vi "Ball Posession Status.vi"(7 "Override?":bool, 9 "Logical Exit?":bool, 10 "Using Sensor?":bool, 11 "Sensor":bool) -> (3 "Ball Posessed?":bool)   [LabVIEW 2015]
uses:
  Common Code/Change Detect Boolean.vi
panel:
  in  "Override to True?":bool
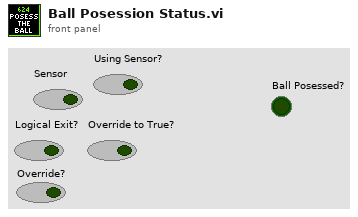
[diagram p1: front panel]
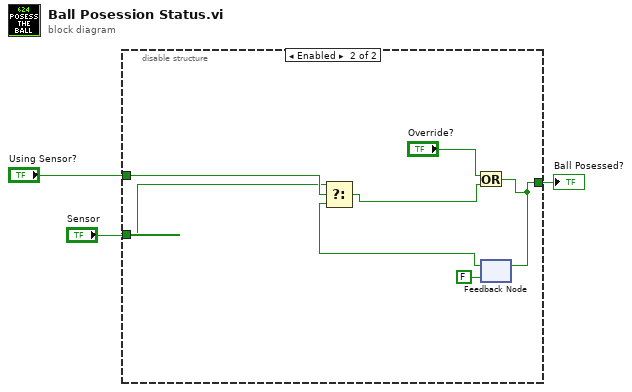
[diagram p0: block diagram]
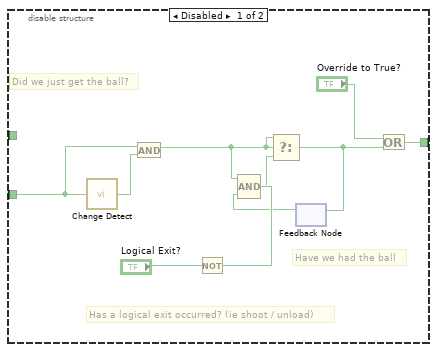
[diagram p2: hidden frame]
diagram:
  n1 = disable-structure shown="Enabled" {
    disable-tunnel: "Sensor" -> [w12 w19]
    disable-tunnel: [w6 w14] -> w2
    disable-tunnel: "Using Sensor?" -> [_ w20]
    frame Disabled {
      # "Has a logical exit occurred? (ie shoot / unload)"
      # "Have we had the ball"
      # "Did we just get the ball?"
      n2 = call-poly "Change Detect.vi"("In"=w12) -> ("Changed?"=w13:bool)
      n3 = And(x=w12, y=w13) -> (x .and. y?=w4:bool)
      n4 = Not(x="Logical Exit?") -> (.not. x?=w10:bool)
      n5 = feedback #1() -> (w9:bool)  [unwired: 1 in]
      n6 = Compound Arithmetic op=AND(w4, w10, w9) -> (w8:bool)
      n7 = Select(t=w4, s=w4, f=w8) -> (s? t:f=w7:bool)
      n8 = feedback-in #1(w7) -> ()
      n9 = Or(x="Override to True?", y=w7) -> (x .or. y?=w6:bool)
    }
    frame Enabled {
      n10 = feedback #2(FALSE ("Sensor")) -> (w17:bool)
      n11 = Select(t=w19, s=w20, f=w17) -> (s? t:f=w15:bool)
      n12 = Or(x="Override?", y=w15) -> (x .or. y?=w14:bool)
      n13 = feedback-in #2(w14) -> ()
    }
  }
  "Ball Posessed?" <- w2
